vi "testPythonCompiler.vi"() -> ()   [LabVIEW 2011, in "run.lvlib"]
uses:
  run.lvlib
panel:
  out "Devices":string[](array[string])
  out "output":string
  in  "scriptPath":path=path "C:/Users/Administrator/Desktop/Crete/Data/Scripts/ScriptRunFolder/141114_0031_03 06Amp-Dimple-CB3-CB2-CB1-CB4-LR_Dp.xml"
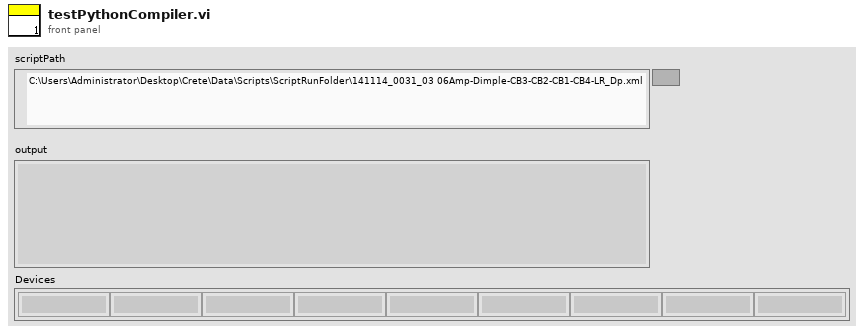
[diagram p1: front panel]
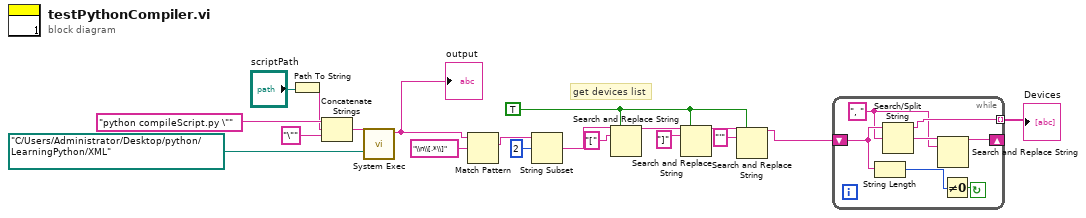
[diagram p0: block diagram]
diagram:
  w6 = TRUE ("replace all? (F)")
  # "get devices list"
  n1 = Path To String(path="scriptPath") -> (string=w16:string)
  n2 = Concatenate Strings("python compileScript.py \"", w16, "\"") -> (w15:string)
  n3 = call <vilib>:"System Exec.vi"("working directory"=path "C:/Users/Administrator/Desktop/python/LearningPython/XML", "command line"=w15) -> ("standard output"=w13:string)  [unwired: 6 in, 3 out]
  "output" <- w13
  n4 = Match Pattern(string=w13, regular expression="\\n\\[.*\\]") -> (match substring=w5:string)  [unwired: 1 in, 3 out]
  n5 = String Subset(string=w5, offset (0)=2) -> (substring=w3:string)  [unwired: 1 in]
  n6 = Search and Replace String(replace all?=w6, input string=w3, search string="[") -> (result string=w10:string)  [unwired: 5 in, 3 out]
  n7 = Search and Replace String(replace all?=w6, input string=w10, search string="]") -> (result string=w8:string)  [unwired: 5 in, 3 out]
  n8 = Search and Replace String(replace all?=w6, input string=w8, search string="'") -> (result string=w2:string)  [unwired: 5 in, 3 out]
  n9 = while {
    shift-right: [w20] -> _
    shift-left: w2 -> [w24]
    tunnel: [w23] -> w1 mode=indexing
    stop <- w26 continue-if-true
    w21 = ", " ("search string/char (-)")
    n10 = String Length(string=w24) -> (length=w25:i32)
    n11 = Search/Split String(string=w24, search string/char (-)=w21) -> (substring before match=w23:string, match + rest of string=w22:string)  [unwired: 1 in, 1 out]
    n12 = Search and Replace String(input string=w22, search string=w21) -> (result string=w20:string)  [unwired: 6 in, 3 out]
    n13 = Not Equal To 0?(x=w25) -> (x != 0?=w26:bool)
  }
  "Devices" <- w1
